vi "Start Window Drag.vi"(8 "error in (no error)":errorcluster, 11 "VI Ref (calling VI)":refnum<vi>) -> (0 "error out":errorcluster, 3 "dup VI Ref":refnum<vi>)   [LabVIEW 2021]
uses:
  user32.dll
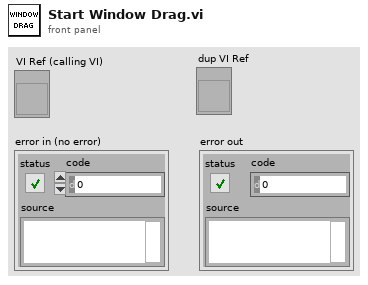
[diagram p1: front panel]
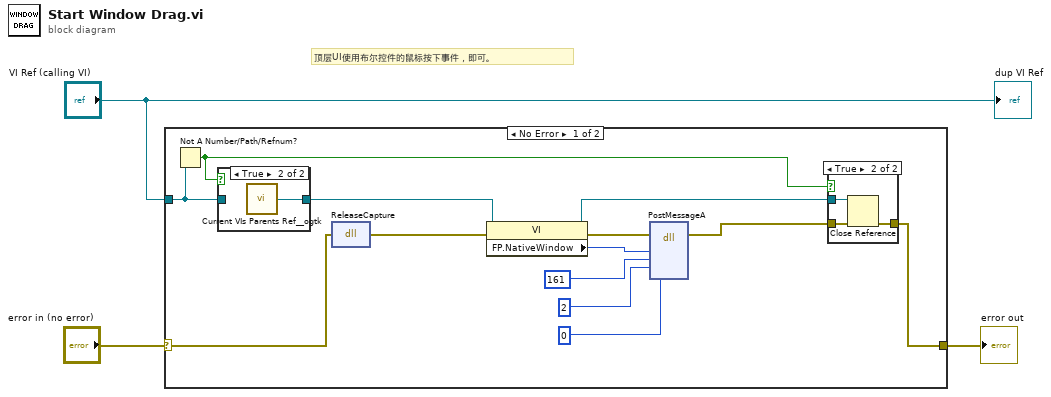
[diagram p0: block diagram]
diagram:
  # "顶层UI使用布尔控件的鼠标按下事件，即可。"
  n1 = case shown="No Error" "error in (no error)" {
    selector: "error in (no error)" -> [w16 w23]
    tunnel: "VI Ref (calling VI)" -> [w9 _]
    tunnel: [w4 w23] -> w3
    frame No Error {
      n2 = Not A Number/Path/Refnum?(number/path/refnum=w9) -> (NaN/Path/Refnum?=w8:bool)
      n3 = case shown="True" w8 {
        tunnel: [w21 w22] -> w7
        tunnel: w9 -> [w21 _]
        frame False {
        }
        frame True {
          n4 = call <userlib>:"Current VIs Parents Ref__ogtk.vi"() -> ("Calling VI's Reference"=w22:refnum<vi>)  [unwired: 2 in]
        }
      }
      n5 = dll-call lib="user32.dll" fn="ReleaseCapture"(error in=w16) -> (error out=w15:errorcluster)  [unwired: 3 in, 1 out]
      n6 = property class="VI"(reference=w7, error in=w15) -> (reference out=w6:refnum<vi>, error out=w14:errorcluster, "FP.NativeWindow"=w13:u64)
      n7 = dll-call lib="user32.dll" fn="PostMessageA"(error in=w14, "hWnd"=w13, "Msg"=161, "wParam"=2, "lParam"=0) -> (error out=w5:errorcluster)  [unwired: 7 in, 1 out]
      n8 = case shown="True" w8 {
        tunnel: w6 -> [_ w20]
        tunnel: w5 -> [w17 w19]
        tunnel: [w17 w18] -> w4
        frame False {
        }
        frame True {
          n9 = Close Reference(reference=w20, error in (no error)=w19) -> (error out=w18:errorcluster)
        }
      }
    }
    frame Error {
    }
  }
  "error out" <- w3
  "dup VI Ref" <- "VI Ref (calling VI)"
